vi "Temperature Controller Main.vi"() -> ()   [LabVIEW 2016, in "Desktop Application.lvlib"]
uses:
  Desktop Application.lvlib
  <vilib>/Skyline/Message/HTTP Wrapper/NI Skyline Message HTTP.lvclass
  <vilib>/Skyline/Configuration/Configuration HTTP_class/NI Skyline Configuration HTTP.lvclass
  <vilib>/Skyline/Configuration/Configuration HTTP_class/Open Configuration HTTP.vi
  <vilib>/Skyline/Message/HTTP Wrapper/Open (HTTP).vi
  <vilib>/Skyline/Message/NI Skyline Message.lvclass
  <vilib>/Skyline/Configuration/Configuration_class/NI Skyline Configuration.lvclass
panel:
  out "Heater State":bool
  in  "Low Limit":dbl
  in  "High Limit":dbl
  in  "Programatic Stop":bool
  out "CurrentTemperature":dbl(slide) scale=0.0..100.0
  out "Heater State Trend":i16(graph)
  out "Temperature Trend":T1(graph)
  # "Temperature Controller running on windows"
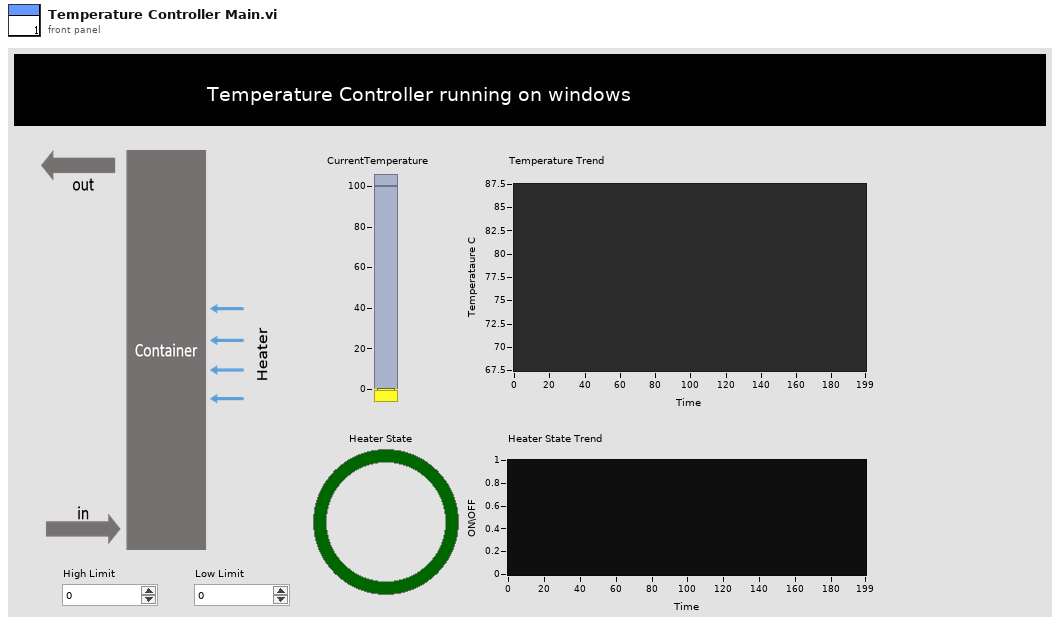
[diagram p1: front panel]
types:
  T1 = cluster{"Current Temp":dbl, "Low Set Point":dbl, "High Set Point":dbl}
  T2 = enum32{"invalid app kind", "Development System", "Run Time System", "Student Edition", "Embedded LabVIEW", "Evaluation", "Custom"}
  T3 = cluster{"Current Temp":dbl, "Low Set Point":dbl, "High Set Point":dbl}[]
  T4 = enum32{"Invalid", "Standard", "Closed", "Hidden", "Minimized", "Maximized"}
  T5 = cluster{"Core":cluster{"Current VI Reference":refnum<vi>, "Close Panel on Exit?":bool}, "High Set Point":dbl, "Low Set Point":dbl, "Current Temp":dbl, "Heater ON?":bool, "Skyline":refnum<class "NI Skyline Message HTTP.lvclass">, "SLconnected?":bool, "HTTP onfiguration":refnum<class "NI Skyline Configuration HTTP.lvclass">}
  T6 = cluster{"Current VI Reference":refnum<vi>, "Close Panel on Exit?":bool}
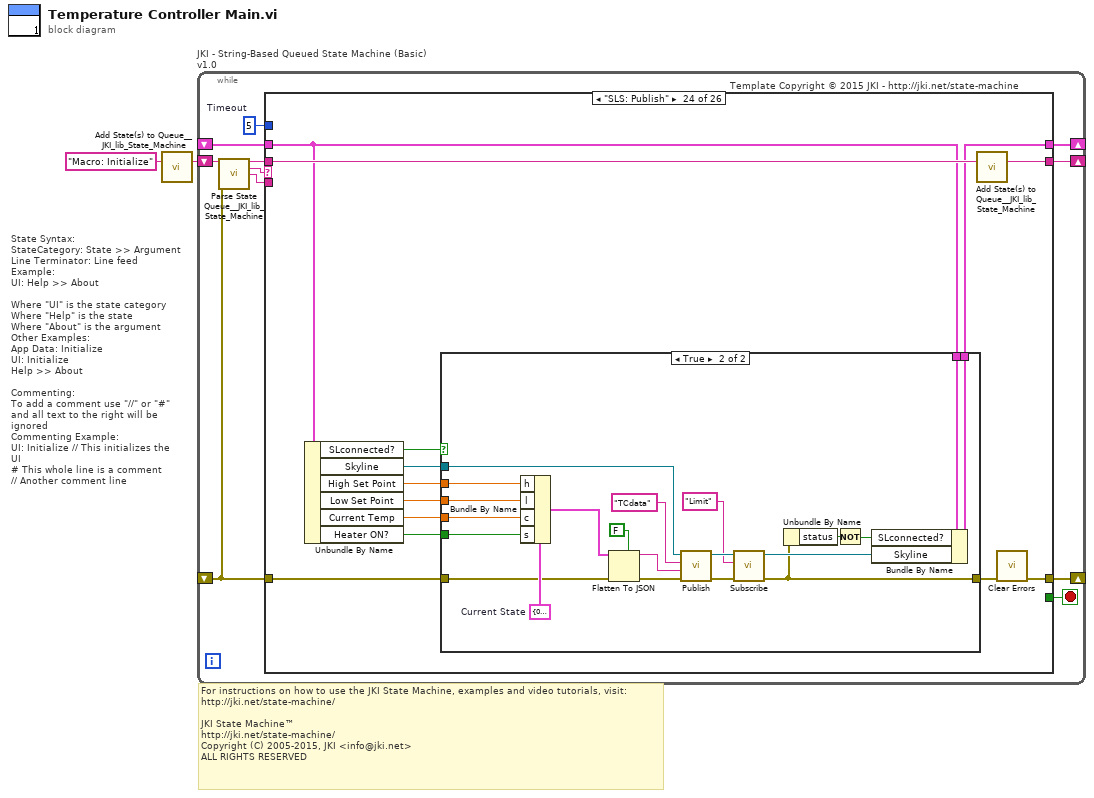
[diagram p0: block diagram]
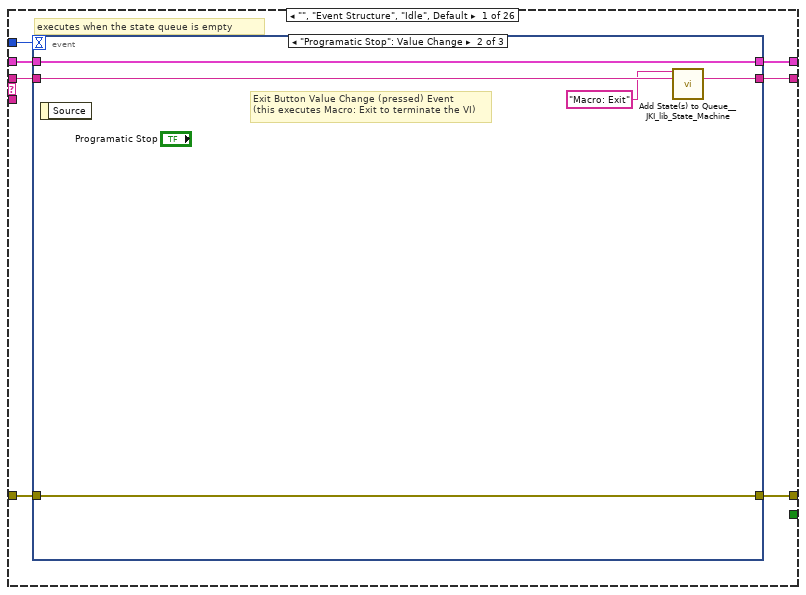
[diagram p2: hidden frame]
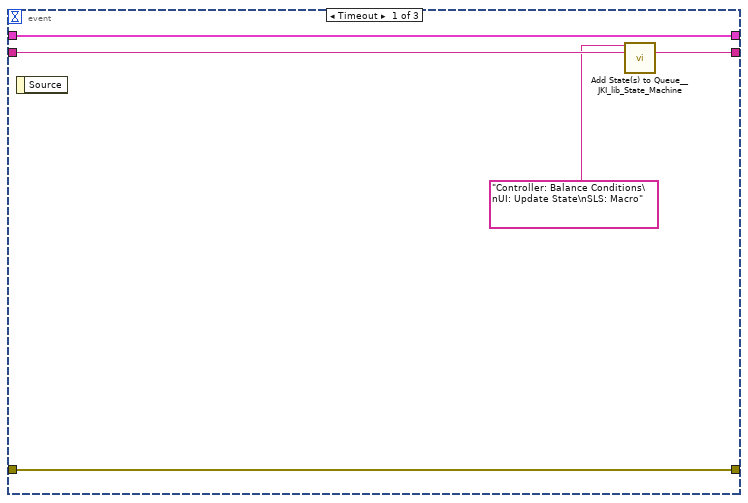
[diagram p3: hidden frame]
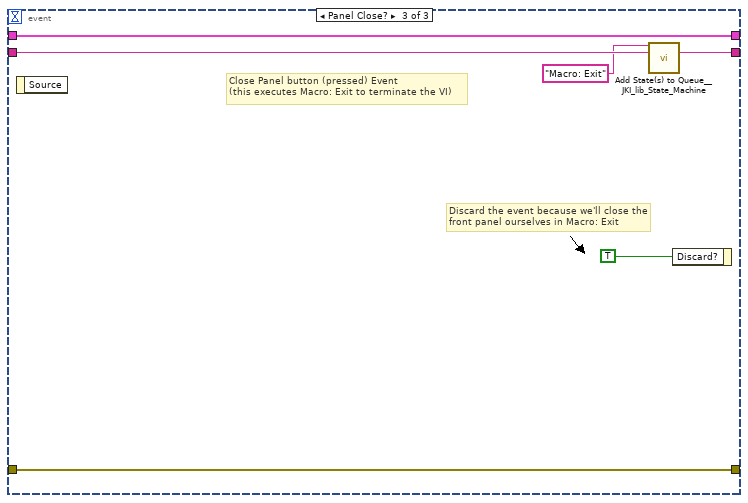
[diagram p4: hidden frame]
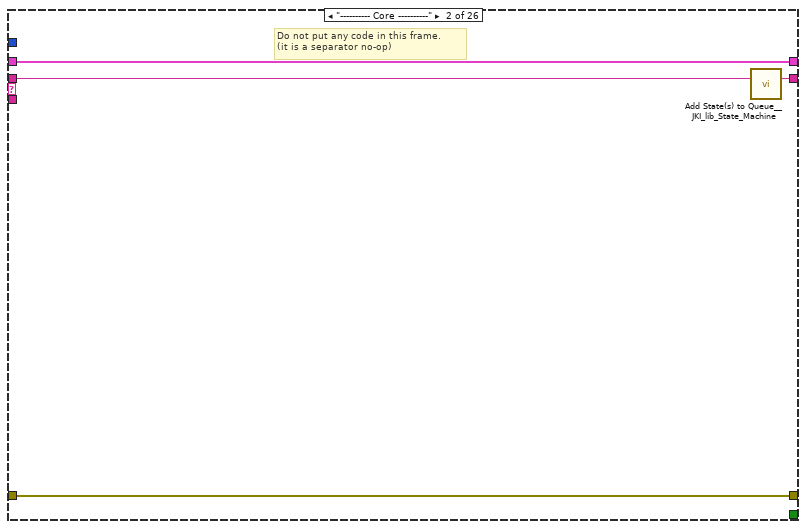
[diagram p5: hidden frame]
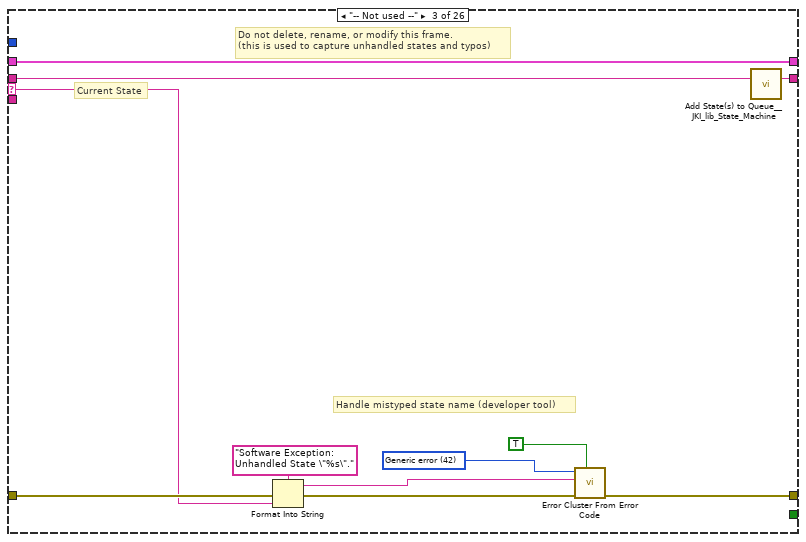
[diagram p6: hidden frame]
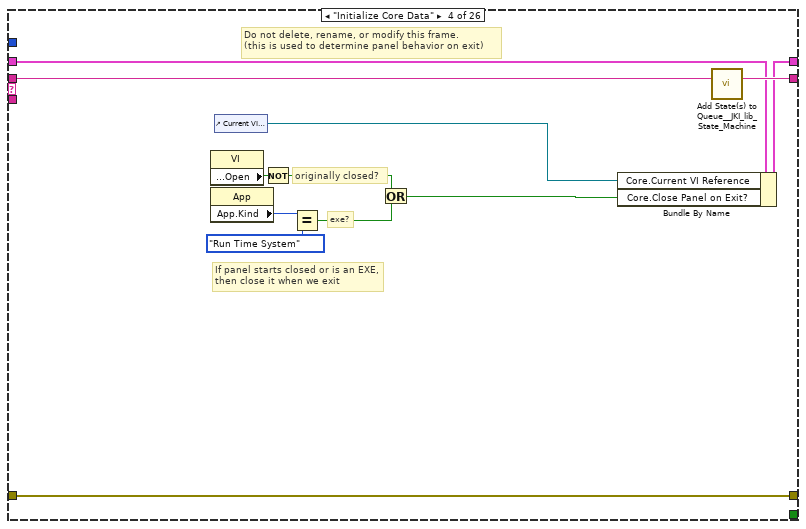
[diagram p7: hidden frame]
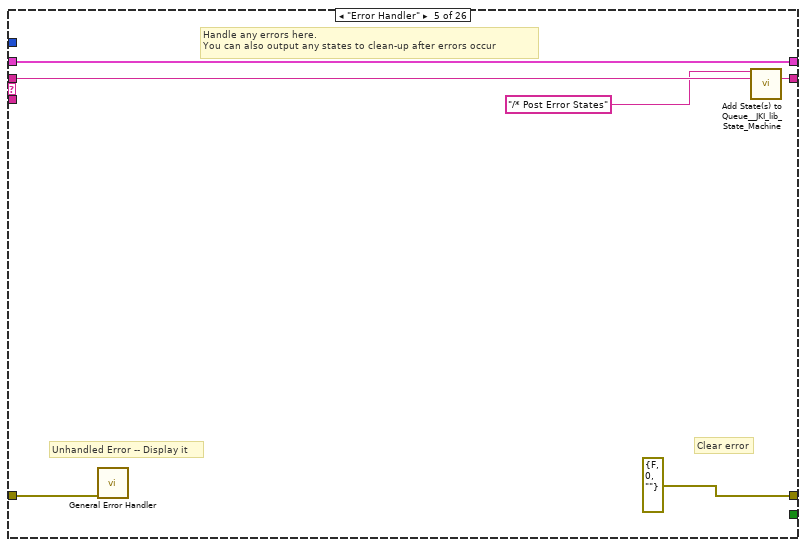
[diagram p8: hidden frame]
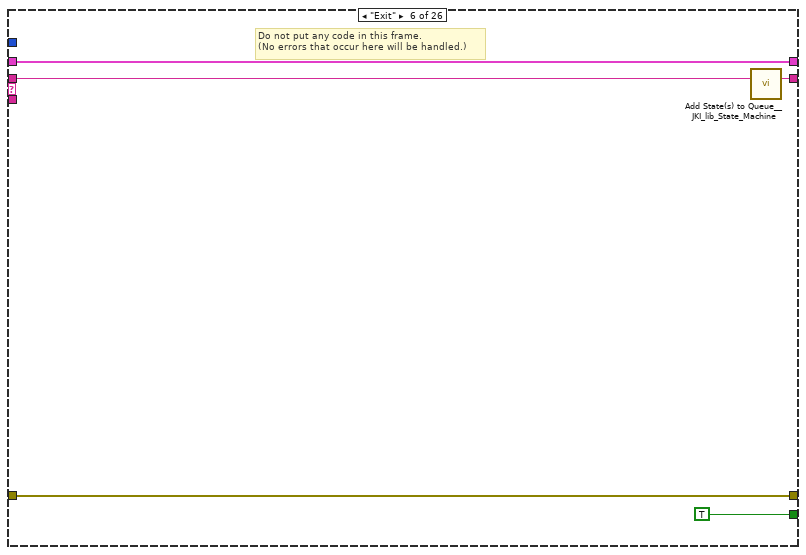
[diagram p9: hidden frame]
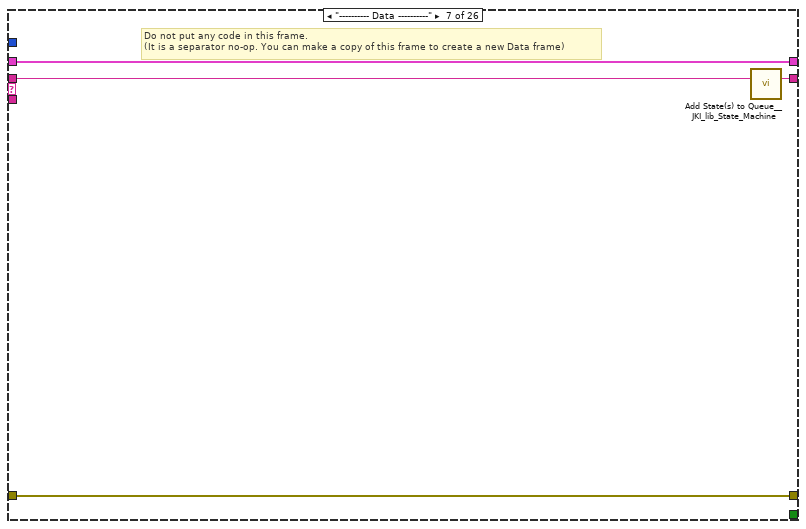
[diagram p10: hidden frame]
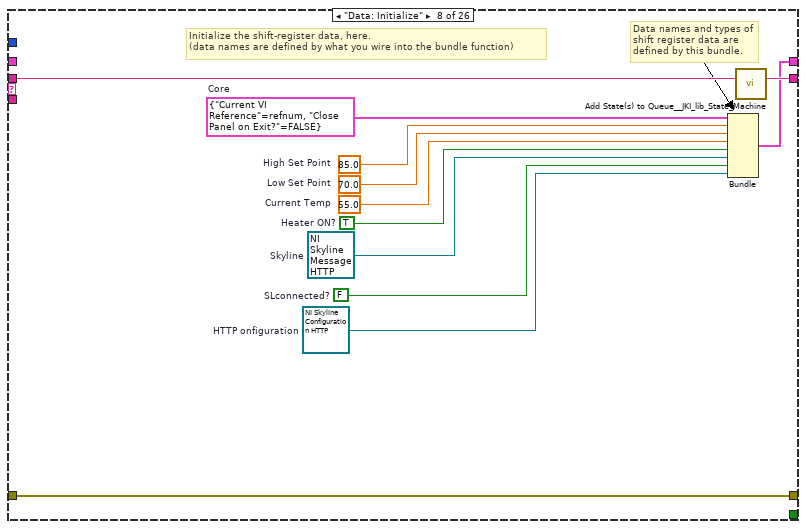
[diagram p11: hidden frame]
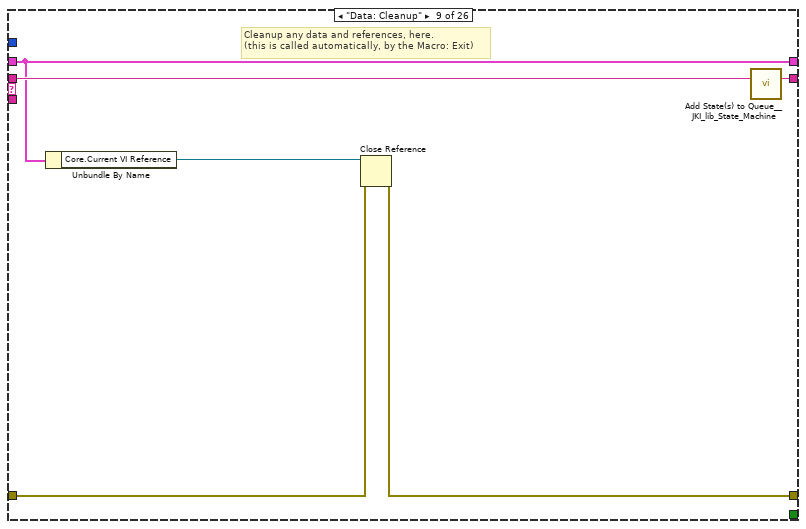
[diagram p12: hidden frame]
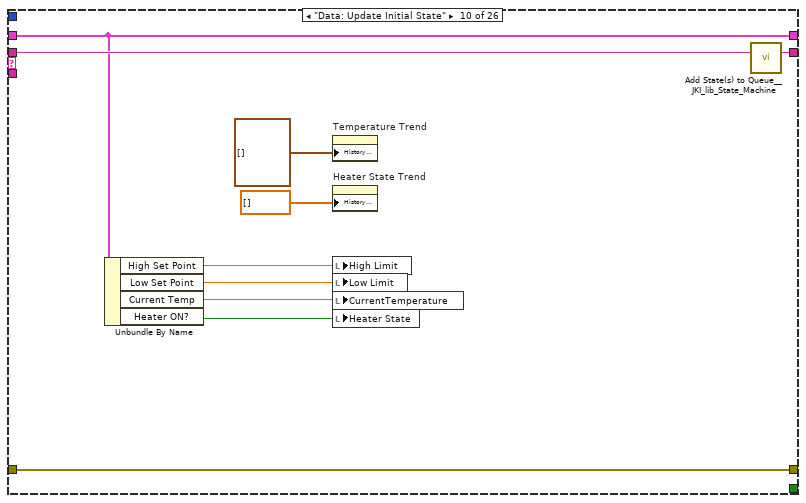
[diagram p13: hidden frame]
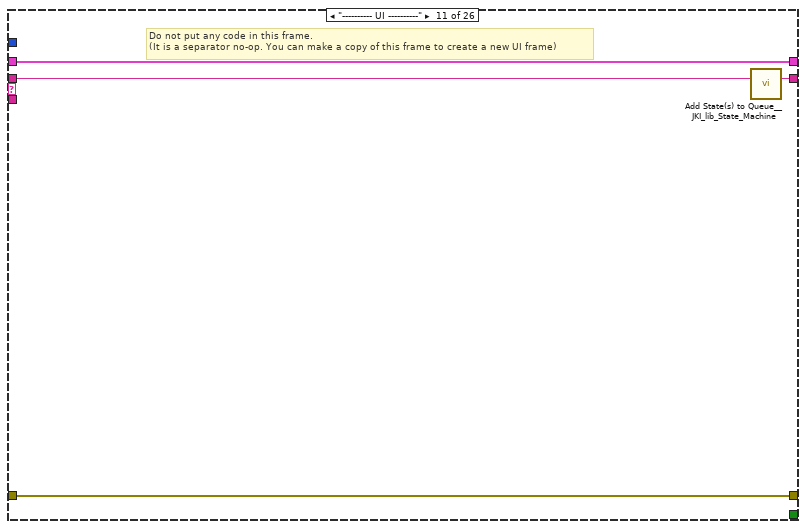
[diagram p14: hidden frame]
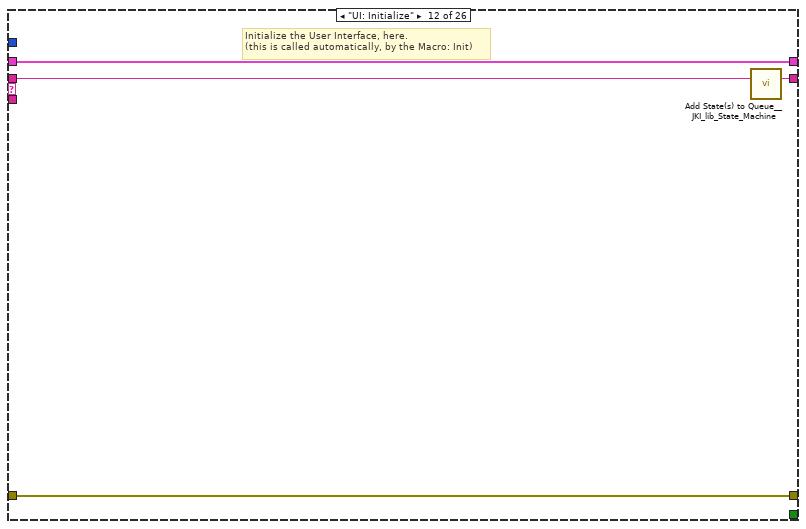
[diagram p15: hidden frame]
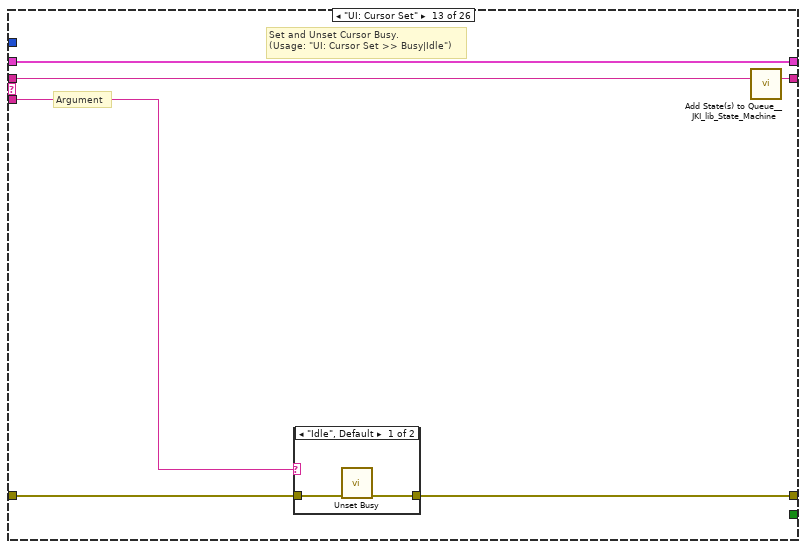
[diagram p16: hidden frame]
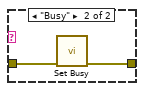
[diagram p17: hidden frame]
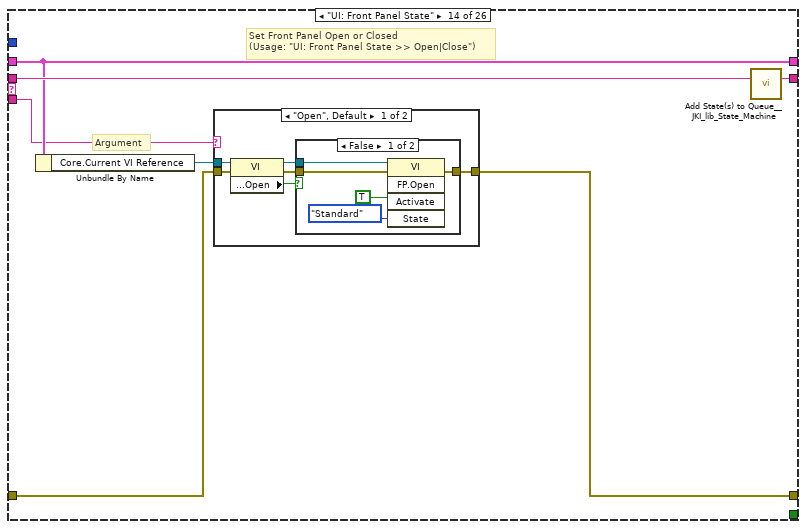
[diagram p18: hidden frame]
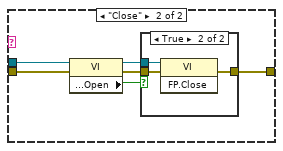
[diagram p20: hidden frame]
diagram:
  # "For instructions on how to use the JKI State Machine, examples and video tutorials, visit:\nhttp://jki.net/state-machine/\n\nJKI State Machine™\nhttp://jki.net/state-machine/\nCopyright (C) 2005-2015, JKI <info@jki.net>\nALL RIGHTS RESERVED"
  # "State Syntax:\nStateCategory: State >> Argument\nLine Terminator: Line feed\nExample:\nUI: Help >> About\n\nWhere \"UI\" is the state category\nWhere \"Help\" is the state\nWhere \"About\" is the argument\nOther Examples:\nApp Data: Initialize\nUI: Initialize\nHelp >> About\n\nCommenting:\nTo add a comment use \"//\" or \"#\" and all text to the right will be ignored\nCommenting Example:\nUI: Initialize // This initializes the UI\n# This whole line is a comment\n// Another comment line"
  n1 = call <vilib>:"Add State(s) to Queue__JKI_lib_State_Machine.vi"("State(s) in (\"\")"="Macro: Initialize") -> ("States Out"=w2:string)  [unwired: 14 in]
  n2 = while "JKI - String-Based Queued State Machine (Basic) v1.0" {
    shift-right: [w6] -> _
    shift-left: _ -> [w5]
    shift-right: [w9] -> _
    shift-left: _ -> [w3]
    shift-right: [w8] -> _
    shift-left: w2 -> [w10]
    stop <- w7 stop-if-true
    w4 = 5  # Timeout
    # "Template Copyright © 2015 JKI - http://jki.net/state-machine"
    n3 = call <vilib>:"Parse State Queue__JKI_lib_State_Machine.vi"("State Queue"=w10, "Error In (no error)"=w3) -> ("Remaining States"=w12:string, "Current State"=w13:string, "Arguments"=w11:string)  [unwired: 11 in]
    n4 = case shown="\"SLS: Publish\"" w13 {
      selector: w13 -> [_ _ w41 _ _ _ _ _ _ _ _ _ _ _ _ _ _ _ _ _ _ _ _ _ _ _]
      tunnel: w12 -> [w20 w40 w45 w63 w69 w74 w78 w90 w96 w106 w110 w114 w120 w131 w162 w167 w172 w177 w187 w191 w209 w211 w219 w246 w273 w299]
      tunnel: w11 -> [_ _ _ _ _ _ _ _ _ _ _ _ w115 w125 _ _ _ _ _ _ _ _ _ _ _ _]
      tunnel: w5 -> [w18 w37 w43 w54 w66 w72 w75 _ w91 w101 w107 w112 w118 w127 w160 w164 w169 w174 w184 w188 w204 w212 w216 w236 w274 w298]
      tunnel: [w17 w38 w47 w60 errorcluster {"status"=FALSE, "code"=0, "source"=""} ("error out") w71 w76 w87 w92 w104 w108 w111 w116 w128 w163 w165 w170 w175 w185 w189 w207 w210 w214 w239 w270 w295] -> w9
      tunnel: w3 -> [w16 w38 w46 w60 w65 w71 w76 w87 w93 w104 w108 w111 w117 w129 w163 w165 w170 w175 w185 w189 w207 w210 w218 w240 w275 w296]
      tunnel: [w19 w39 w44 w62 w68 w73 w77 w89 w95 w105 w109 w113 w119 w130 w161 w166 w171 w176 w186 w190 w208 w211 w219 w245 w273 w299] -> w8
      tunnel: [_ _ _ _ _ TRUE _ _ _ _ _ _ _ _ _ _ _ _ _ _ _ _ _ _ _ _] -> w7
      tunnel: [w15 w37 w43 w61 w66 w72 w75 w88 w91 w101 w107 w112 w118 w127 w160 w164 w169 w174 w184 w188 w203 w212 w217 w235 w274 w298] -> w6
      tunnel: w4 -> [w14 _ _ _ _ _ _ _ _ _ _ _ _ _ _ _ _ _ _ _ _ _ _ _ _ _]
      frame "", "Event Structure", "Idle", Default {
        # "executes when the state queue is empty"
        n5 = event shown="[1] \"Programatic Stop\": Value Change" {
          selector: _ -> [_ _ _]
          dyn-events: _ -> [_ _ _]
          timeout: w14 -> [_ _ _]
          tunnel: w20 -> [w25 w30 w36]
          tunnel: [w24 w29 w35] -> w19
          tunnel: w18 -> [w22 w27 w33]
          tunnel: [w23 w28 w34] -> w17
          tunnel: w16 -> [w23 w28 w34]
          tunnel: [w22 w27 w33] -> w15
          event Timeout {
            n6 = event-data() -> ()  [unwired: 1 in, 1 out]
            n7 = call <vilib>:"Add State(s) to Queue__JKI_lib_State_Machine.vi"("State(s) in Front (\"\")"="Controller: Balance Conditions\nUI: Update State\nSLS: Macro" ("State(s) in Front (\"\")"), "State(s) in (\"\")"=w25) -> ("States Out"=w24:string)  [unwired: 13 in]
          }
          event "Programatic Stop": Value Change {
            # "Exit Button Value Change (pressed) Event\n(this executes Macro: Exit to terminate the VI)"
            n8 = event-data() -> ()  [unwired: 1 in, 1 out]
            n9 = call <vilib>:"Add State(s) to Queue__JKI_lib_State_Machine.vi"("State(s) in Front (\"\")"="Macro: Exit", "State(s) in (\"\")"=w30) -> ("States Out"=w29:string)  [unwired: 13 in]
          }
          event Panel Close? {
            # "Discard the event because we'll close the front panel ourselves in Macro: Exit"
            # "Close Panel button (pressed) Event\n(this executes Macro: Exit to terminate the VI)"
            n10 = event-data() -> ()  [unwired: 1 in, 1 out]
            n11 = call <vilib>:"Add State(s) to Queue__JKI_lib_State_Machine.vi"("State(s) in Front (\"\")"="Macro: Exit", "State(s) in (\"\")"=w36) -> ("States Out"=w35:string)  [unwired: 13 in]
            n12 = event-data("Discard?"=TRUE) -> ()  [unwired: 1 in, 1 out]
          }
        }
      }
      frame "---------- Core ----------" {
        # "Do not put any code in this frame.\n(it is a separator no-op)"
        n13 = call <vilib>:"Add State(s) to Queue__JKI_lib_State_Machine.vi"("State(s) in (\"\")"=w40) -> ("States Out"=w39:string)  [unwired: 14 in]
      }
      frame "-- Not used --" {
        w50 = 42 items=["No error", "Argument error", "Memory is full", "Out of zone", "End of file", "File already open", "Generic file I/O error", "File not found", "File permission error", "Disk is full", "Duplicate path", "Too many files open", "System feature not enabled", "Resource file not found", "Cannot add resource", "Resource not found", "Image not found", "Image memory error", "Pen does not exist", "Config type invalid", "Config token not found", "Config parse error", "Config memory error", "Bad external code format", "Bad external code offset", "External code not present", "Null window", "Destroy window error", "Null menu", "Print aborted", "Bad print record", "Print driver error", "Windows error during printing", "Memory error during printing", "Print dialog error", "Generic print error", "Invalid device refnum", "Device not found", "Device parameter error", "Device unit error", "Cannot open device", "Device call aborted", "Generic error", "Cancelled by user", "Object ID too low", "Object ID too high", "Object not in heap", "Unknown heap", "Unknown object (invalid DefProc)", "Unknown object (DefProc not in table)", "Message out of range", "Invalid (null) method", "Unknown message", "Manager call not supported", "Bad address", "Network operation in progress", "Network operation timed out", "Connection is busy", "Network attribute not supported", "Network error", "Address in use", "System out of memory", "Connection aborted", "Connection refused", "Not connected", "Already connected", "Connection closed", "Initialization error (interapplication manager)", "Bad occurrence", "Wait on unbound occurrence handler", "Occurrence queue overflow", "Datalog type conflict", "Unused", "Unrecognized type (interapplication manager)", "Memory corrupt", "Failed to make temporary DLL", "Old CIN version", "Drag socket not found", "Failed to load drop-object", "Failed to register OLE object", "Failed to release OLE object", "Format specifier type mismatch", "Unknown format specifier", "Too few format specifiers", "Too many format specifiers", "Scan failed", "Newer CIN version", "Error converting to variant", "Runtime menu error", "Password tampered", "Variant attribute not found", "Incompatible variant data type", "Event data is not available", "Event Store is not present", "Occurrence is not found", "Event Queue is not created", "Event info is not available", "Refnum passed is NULL", "Error retrieving Class GUID", "Error retrieving CoClass GUID", "Error retrieving TypeLib GUID.", "Bad built application magic bytes.", "Specific driver is different from the specific driver associated with the Logical Name.", "There is no session opened to the class driver.", "Max Error", "MAX - Error with config objects", "MAX - Error loading configuration", "MAX - Group not supported"]
        # "Current State"
        # "Do not delete, rename, or modify this frame.\n(this is used to capture unhandled states and typos)"
        # "Handle mistyped state name (developer tool)"
        n14 = Format Into String(format string="Software Exception: Unhandled State \"%s\"." ("message"), error in=w46, w41) -> (resulting string=w49:string, error out=w48:errorcluster)  [unwired: 1 in]
        n15 = call <vilib>:"Error Cluster From Error Code.vi"("show call chain? (False)"=TRUE, "error in (no error)"=w48, "error message (\"\")"=w49, "error code (0)"=w50) -> ("error out"=w47:errorcluster)  [unwired: 5 in]
        n16 = call <vilib>:"Add State(s) to Queue__JKI_lib_State_Machine.vi"("State(s) in (\"\")"=w45) -> ("States Out"=w44:string)  [unwired: 14 in]
      }
      frame "Initialize Core Data" {
        # "Do not delete, rename, or modify this frame.\n(this is used to determine panel behavior on exit)"
        # "originally closed?"
        # "exe?"
        # "If panel starts closed or is an EXE, then close it when we exit"
        n17 = property class="VI"() -> ("Front Panel.Open"=w59:bool)  [unwired: 2 in, 2 out]
        n18 = property class="App"() -> ("App.Kind"=w58:T2)  [unwired: 2 in, 2 out]
        n19 = control-ref of="Current VI Reference"() -> (w52:refnum<vi>)
        n20 = Not(x=w59) -> (.not. x?=w56:bool)
        n21 = Equal?(x=w58, y=T2."Run Time System" ("Application:Kind")) -> (x = y?=w55:bool)
        n22 = Or(x=w56, y=w55) -> (x .or. y?=w53:bool)
        n23 = Bundle By Name(cluster=w54, "Core.Current VI Reference"=w52, "Core.Close Panel on Exit?"=w53) -> (w61:T5)
        n24 = call <vilib>:"Add State(s) to Queue__JKI_lib_State_Machine.vi"("State(s) in (\"\")"=w63) -> ("States Out"=w62:string)  [unwired: 14 in]
      }
      frame "Error Handler" {
        # "Unhandled Error -- Display it"
        # "Handle any errors here.\nYou can also output any states to clean-up after errors occur"
        # "Clear error"
        n25 = call <vilib>:"General Error Handler.vi"("error in (no error)"=w65) -> ()  [unwired: 10 in, 5 out]
        n26 = call <vilib>:"Add State(s) to Queue__JKI_lib_State_Machine.vi"("State(s) in Front (\"\")"="/* Post Error States", "State(s) in (\"\")"=w69) -> ("States Out"=w68:string)  [unwired: 13 in]
      }
      frame "Exit" {
        # "Do not put any code in this frame.\n(No errors that occur here will be handled.)"
        n27 = call <vilib>:"Add State(s) to Queue__JKI_lib_State_Machine.vi"("State(s) in (\"\")"=w74) -> ("States Out"=w73:string)  [unwired: 14 in]
      }
      frame "---------- Data ----------" {
        # "Do not put any code in this frame.\n(It is a separator no-op. You can make a copy of this frame to create a new Data frame)"
        n28 = call <vilib>:"Add State(s) to Queue__JKI_lib_State_Machine.vi"("State(s) in (\"\")"=w78) -> ("States Out"=w77:string)  [unwired: 14 in]
      }
      frame "Data: Initialize" {
        w79 = refnum<class "NI Skyline Configuration HTTP.lvclass"> refnum  # HTTP onfiguration
        w80 = FALSE  # SLconnected?
        w81 = refnum<class "NI Skyline Message HTTP.lvclass"> refnum  # Skyline
        w82 = TRUE  # Heater ON?
        w83 = 55.0  # Current Temp
        w84 = 70.0  # Low Set Point
        w85 = 85.0  # High Set Point
        w86 = T6 {"Current VI Reference"=refnum, "Close Panel on Exit?"=FALSE}  # Core
        # "Data names and types of shift register data are defined by this bundle."
        # "Initialize the shift-register data, here.\n(data names are defined by what you wire into the bundle function)"
        n29 = Bundle("Core"=w86, "High Set Point"=w85, "Low Set Point"=w84, "Current Temp"=w83, "Heater ON?"=w82, "Skyline"=w81, "SLconnected?"=w80, "HTTP onfiguration"=w79) -> (w88:T5)  [unwired: 1 in]
        n30 = call <vilib>:"Add State(s) to Queue__JKI_lib_State_Machine.vi"("State(s) in (\"\")"=w90) -> ("States Out"=w89:string)  [unwired: 14 in]
      }
      frame "Data: Cleanup" {
        # "Cleanup any data and references, here.\n(this is called automatically, by the Macro: Exit)"
        n31 = Unbundle By Name(w91) -> ("Core.Current VI Reference"=w94:refnum<vi>)
        n32 = Close Reference(reference=w94, error in (no error)=w93) -> (error out=w92:errorcluster)
        n33 = call <vilib>:"Add State(s) to Queue__JKI_lib_State_Machine.vi"("State(s) in (\"\")"=w96) -> ("States Out"=w95:string)  [unwired: 14 in]
      }
      frame "Data: Update Initial State" {
        n34 = Unbundle By Name(w101) -> ("High Set Point"=w100:dbl, "Low Set Point"=w99:dbl, "Current Temp"=w97:dbl, "Heater ON?"=w98:bool)
        n35 = property on="Temperature Trend" class="WFChart (strict)"("History Data"=T3 []) -> ()  [unwired: 2 in, 2 out]
        n36 = property on="Heater State Trend" class="WFChart (strict)"("History Data"=dbl[] []) -> ()  [unwired: 2 in, 2 out]
        n37 = local write "High Limit"(w100) -> ()
        n38 = local write "Low Limit"(w99) -> ()
        n39 = local write "CurrentTemperature"(w97) -> ()
        n40 = local write "Heater State"(w98) -> ()
        n41 = call <vilib>:"Add State(s) to Queue__JKI_lib_State_Machine.vi"("State(s) in (\"\")"=w106) -> ("States Out"=w105:string)  [unwired: 14 in]
      }
      frame "---------- UI ----------" {
        # "Do not put any code in this frame.\n(It is a separator no-op. You can make a copy of this frame to create a new UI frame)"
        n42 = call <vilib>:"Add State(s) to Queue__JKI_lib_State_Machine.vi"("State(s) in (\"\")"=w110) -> ("States Out"=w109:string)  [unwired: 14 in]
      }
      frame "UI: Initialize" {
        # "Initialize the User Interface, here.\n(this is called automatically, by the Macro: Init)"
        n43 = call <vilib>:"Add State(s) to Queue__JKI_lib_State_Machine.vi"("State(s) in (\"\")"=w114) -> ("States Out"=w113:string)  [unwired: 14 in]
      }
      frame "UI: Cursor Set" {
        # "Argument"
        # "Set and Unset Cursor Busy.\n(Usage: \"UI: Cursor Set >> Busy|Idle\")"
        n44 = case shown="\"Idle\", Default" w115 {
          tunnel: w117 -> [w122 w124]
          tunnel: [w121 w123] -> w116
          frame "Idle", Default {
            n45 = call <vilib>:"Unset Busy.vi"("error in (no error)"=w122) -> ("error out"=w121:errorcluster)  [unwired: 10 in]
          }
          frame "Busy" {
            n46 = call <vilib>:"Set Busy.vi"("error in (no error)"=w124) -> ("error out"=w123:errorcluster)  [unwired: 9 in, 1 out]
          }
        }
        n47 = call <vilib>:"Add State(s) to Queue__JKI_lib_State_Machine.vi"("State(s) in (\"\")"=w120) -> ("States Out"=w119:string)  [unwired: 14 in]
      }
      frame "UI: Front Panel State" {
        # "Argument"
        # "Set Front Panel Open or Closed\n(Usage: \"UI: Front Panel State >> Open|Close\")"
        n48 = Unbundle By Name(w127) -> ("Core.Current VI Reference"=w126:refnum<vi>)
        n49 = case shown="\"Open\", Default" w125 {
          tunnel: w129 -> [w135 w148]
          tunnel: [w137 w149] -> w128
          tunnel: w126 -> [w136 w146]
          frame "Open", Default {
            n50 = property class="VI"(reference=w136, error in=w135) -> (reference out=w133:refnum<vi>, error out=w134:errorcluster, "Front Panel.Open"=w132:bool)
            n51 = case shown="False" w132 {
              tunnel: [w140 w143] -> w137
              tunnel: w134 -> [w139 w143]
              tunnel: w133 -> [w138 _]
              frame False {
                n52 = invoke class="VI" method="FP.Open"(reference=w138, error in=w139, "Activate"=TRUE, "State"=T4."Standard") -> (error out=w140:errorcluster)  [unwired: 1 in, 4 out]
              }
              frame True {
              }
            }
          }
          frame "Close" {
            n53 = property class="VI"(reference=w146, error in=w148) -> (reference out=w145:refnum<vi>, error out=w147:errorcluster, "Front Panel.Open"=w144:bool)
            n54 = case shown="True" w144 {
              tunnel: [w150 w153] -> w149
              tunnel: w147 -> [w150 w152]
              tunnel: w145 -> [_ w151]
              frame False {
              }
              frame True {
                n55 = invoke class="VI" method="FP.Close"(reference=w151, error in=w152) -> (error out=w153:errorcluster)  [unwired: 1 in, 2 out]
              }
            }
          }
        }
        n56 = call <vilib>:"Add State(s) to Queue__JKI_lib_State_Machine.vi"("State(s) in (\"\")"=w131) -> ("States Out"=w130:string)  [unwired: 14 in]
      }
      frame "UI: Update State" {
        n57 = Unbundle By Name(w160) -> ("High Set Point"=w155:dbl, "Low Set Point"=w156:dbl, "Current Temp"=w157:dbl, "Heater ON?"=w158:bool)
        "CurrentTemperature" <- w157
        "Heater State" <- w158
        n58 = Boolean To (0,1)(Boolean=w158) -> (0, 1=→"Heater State Trend":i16)
        n59 = Bundle("Current Temp"=w157, "Low Set Point"=w156, "High Set Point"=w155) -> (→"Temperature Trend":T1)  [unwired: 1 in]
        n60 = call <vilib>:"Add State(s) to Queue__JKI_lib_State_Machine.vi"("State(s) in (\"\")"=w162) -> ("States Out"=w161:string)  [unwired: 14 in]
      }
      frame "---------- Macro ----------" {
        # "Do not put any code in this frame.\n(It is a separator no-op. You can make a copy of this frame to create a new Macro frame)"
        n61 = call <vilib>:"Add State(s) to Queue__JKI_lib_State_Machine.vi"("State(s) in (\"\")"=w167) -> ("States Out"=w166:string)  [unwired: 14 in]
      }
      frame "Macro: Initialize" {
        w168 = "Data: Initialize\nInitialize Core Data\nUI: Initialize\nUI: Front Panel State >> Open\nData: Update Initial State\nUI: Update State\nSLS: Open"  # Data: Initialize Initialize Core Data UI: Initialize UI: Front Panel State >> Open Data: Update Initial State UI: Update State SLS: Open
        # "Initialization Macro\n(This is called once, when the VI starts)"
        n62 = call <vilib>:"Add State(s) to Queue__JKI_lib_State_Machine.vi"("State(s) in Front (\"\")"=w168, "State(s) in (\"\")"=w172) -> ("States Out"=w171:string)  [unwired: 13 in]
      }
      frame "SLS: Macro" {
        # "Initialization Macro\n(This is called once, when the VI starts)"
        n63 = call <vilib>:"Add State(s) to Queue__JKI_lib_State_Machine.vi"("State(s) in Front (\"\")"="SLS: Open\nSLS: Publish\nSLS: Read", "State(s) in (\"\")"=w177) -> ("States Out"=w176:string)  [unwired: 13 in]
      }
      frame "Macro: Exit" {
        # "Exit Macro\n(This is called once, when the VI exits)"
        n64 = Unbundle By Name(w184) -> ("Core.Close Panel on Exit?"=w183:bool)
        n65 = Select(t="UI: Front Panel State >> Close", s=w183, f="") -> (s? t:f=w180:string)
        n66 = call <vilib>:"Add State(s) to Queue__JKI_lib_State_Machine.vi"("State(s) in (\"\")"=w180, "State(s) at Back (\"\")"="Data: Cleanup\nSLS: Close\nExit") -> ("States Out"=w178:string)  [unwired: 13 in]
        n67 = call <vilib>:"Add State(s) to Queue__JKI_lib_State_Machine.vi"("State(s) in Front (\"\")"=w178, "State(s) in (\"\")"=w187) -> ("States Out"=w186:string)  [unwired: 13 in]
      }
      frame "---------- Functions ----------" {
        # "Template Separator\n(You can make a copy of, or modify, this frame)"
        n68 = call <vilib>:"Add State(s) to Queue__JKI_lib_State_Machine.vi"("State(s) in (\"\")"=w191) -> ("States Out"=w190:string)  [unwired: 14 in]
      }
      frame "Controller: Balance Conditions" {
        n69 = Unbundle By Name(w204) -> ("Heater ON?"=w196:bool, "Current Temp"=w194:dbl)
        n70 = Max & Min(x="High Limit", y="Low Limit") -> (max(x,y)=w202:dbl, min(x,y)=w193:dbl)
        n71 = Less?(x=w194, y=w193) -> (x < y?=w192:bool)
        n72 = In Range and Coerce(upper limit=w202, x=w194, lower limit=w193) -> (In Range?=w197:bool)  [unwired: 1 out]
        n73 = Increment(x=w194) -> (x+1=w200:dbl)
        n74 = Decrement(x=w194) -> (x-1=w201:dbl)
        n75 = Select(t=w196, s=w197, f=w192) -> (s? t:f=w195:bool)
        n76 = Select(t=w200, s=w195, f=w201) -> (s? t:f=w199:dbl)
        n77 = Bundle By Name(cluster=w204, "High Set Point"=w202, "Low Set Point"=w193, "Heater ON?"=w195, "Current Temp"=w199) -> (w203:T5)
        n78 = Wait (ms)(milliseconds to wait=u32 300) -> ()  [unwired: 1 out]
        n79 = call <vilib>:"Add State(s) to Queue__JKI_lib_State_Machine.vi"("State(s) in (\"\")"=w209) -> ("States Out"=w208:string)  [unwired: 14 in]
      }
      frame "----------System Link Service----------" {
      }
      frame "SLS: Open" {
        n80 = Unbundle By Name(w216) -> ("SLconnected?"=w213:bool)
        n81 = case shown="True" w213 {
          tunnel: w218 -> [w231 w232]
          tunnel: [w229 w233] -> w217
          tunnel: w216 -> [w228 w233]
          tunnel: [w227 w232] -> w215
          frame False {
            n82 = call-poly <vilib>:"Open Configuration.vi"("error in (no error)"=w231, "password"="q", "username"="admin", "server url"="http://localhost:80") -> ("error out"=w223:errorcluster, "HTTP configuration out"=w224:refnum<class "NI Skyline Configuration HTTP.lvclass">)  [unwired: 6 in]
            n83 = call-poly <vilib>:"Open.vi"("configuration"=w224, "error in (no error)"=w223) -> ("error out"=w227:errorcluster, "message http out"=w230:refnum<class "NI Skyline Message HTTP.lvclass">)  [unwired: 8 in]
            n84 = Unbundle By Name(w227) -> ("status"=w226:bool)
            n85 = Not(x=w226) -> (.not. x?=w225:bool)
            n86 = Bundle By Name(cluster=w228, "HTTP onfiguration"=w224, "SLconnected?"=w225, "Skyline"=w230) -> (w229:T5)
          }
          frame True {
          }
        }
        n87 = call <vilib>:"Clear Errors.vi"("error in (no error)"=w215) -> ("error out"=w214:errorcluster)  [unwired: 5 in, 1 out]
      }
      frame "SLS: Publish" {
        n88 = Unbundle By Name(w236) -> ("SLconnected?"=w234:bool, "Skyline"=w237:refnum<class "NI Skyline Message HTTP.lvclass">, "High Set Point"=w244:dbl, "Low Set Point"=w243:dbl, "Current Temp"=w242:dbl, "Heater ON?"=w241:bool)
        n89 = case shown="True" w234 {
          tunnel: w244 -> [_ w268]
          tunnel: w243 -> [_ w267]
          tunnel: w242 -> [_ w266]
          tunnel: w241 -> [_ w265]
          tunnel: w240 -> [w248 w263]
          tunnel: [w248 w250] -> w238
          tunnel: w237 -> [_ w260]
          tunnel: w236 -> [w247 w259]
          tunnel: [w247 w258] -> w235
          frame False {
          }
          frame True {
            w269 = cluster{"h":dbl, "l":dbl, "c":dbl, "s":bool} {"h"=0.0, "l"=0.0, "c"=0.0, "s"=FALSE}  # Current State
            n90 = Bundle By Name(cluster=w269, "h"=w268, "l"=w267, "c"=w266, "s"=w265) -> (w264:cluster{"h":dbl, "l":dbl, "c":dbl, "s":bool})
            n91 = Flatten To JSON(enable LabVIEW extensions? (T)=FALSE, anything=w264, error in (no error)=w263) -> (JSON string=w257:string, 11:w261:errorcluster)
            n92 = call-dynamic "Publish.vi"("error in (no error)"=w261, "message"=w257, "topic"="TCdata", "message http"=w260) -> ("error out"=w251:errorcluster, "message http out"=w253:refnum<class "NI Skyline Message HTTP.lvclass">)  [unwired: 6 in]
            n93 = call-dynamic "Subscribe.vi"("error in (no error)"=w251, "topic"="Limit", "message http"=w253) -> ("error out"=w250:errorcluster, "message http out"=w252:refnum<class "NI Skyline Message HTTP.lvclass">)  [unwired: 7 in]
            n94 = Unbundle By Name(w250) -> ("status"=w255:bool)
            n95 = Not(x=w255) -> (.not. x?=w254:bool)
            n96 = Bundle By Name(cluster=w259, "SLconnected?"=w254, "Skyline"=w252) -> (w258:T5)
          }
        }
        n97 = call <vilib>:"Add State(s) to Queue__JKI_lib_State_Machine.vi"("State(s) in (\"\")"=w246) -> ("States Out"=w245:string)  [unwired: 14 in]
        n98 = call <vilib>:"Clear Errors.vi"("error in (no error)"=w238) -> ("error out"=w239:errorcluster)  [unwired: 5 in, 1 out]
      }
      frame "SLS: Read" {
        n99 = Unbundle By Name(w274) -> ("SLconnected?"=w271:bool, "Skyline"=w272:refnum<class "NI Skyline Message HTTP.lvclass">)
        n100 = case shown="True" w271 {
          tunnel: w275 -> [w276 w284]
          tunnel: w272 -> [_ w283]
          tunnel: [w276 w277] -> w270
          frame False {
          }
          frame True {
            n101 = call-dynamic "Read.vi"("error in (no error)"=w284, "timeout milliseconds (100)"=100, "message http"=w283) -> ("error out"=w278:errorcluster, "message"=w279:string, "topic"=w280:string, "dequeue status"=w281:bool)  [unwired: 4 in, 1 out]
            n102 = case shown="True" w281 {
              tunnel: w280 -> [_ _]
              tunnel: w279 -> [_ w290]
              tunnel: w278 -> [w285 w292]
              tunnel: [w285 w291] -> w277
              frame False {
              }
              frame True {
                w289 = cluster{"high":dbl, "low":dbl} {"high"=0.0, "low"=0.0}  # limit
                n103 = Unflatten From JSON(JSON string=w290, type and defaults=w289, error in (no error)=w292) -> (value=w288:cluster{"high":dbl, "low":dbl}, error out=w291:errorcluster)  [unwired: 4 in]
                n104 = Unbundle(w288) -> ("high"=w287:dbl, "low"=w286:dbl)
                n105 = local write "High Limit"(w287) -> ()
                n106 = local write "Low Limit"(w286) -> ()
              }
            }
          }
        }
      }
      frame "SLS: Close" {
        n107 = Unbundle By Name(w298) -> ("HTTP onfiguration"=w293:refnum<class "NI Skyline Configuration HTTP.lvclass">, "SLconnected?"=w294:bool, "Skyline"=w297:refnum<class "NI Skyline Message HTTP.lvclass">)
        n108 = case shown="True" w294 {
          tunnel: w297 -> [_ w303]
          tunnel: w296 -> [w300 w304]
          tunnel: [w300 w306] -> w295
          tunnel: w293 -> [_ w308]
          frame False {
          }
          frame True {
            n109 = call-dynamic "Unsubscribe.vi"("error in (no error)"=w304, "topic"="Limit", "message http"=w303) -> ("error out"=w301:errorcluster, "message http out"=w302:refnum<class "NI Skyline Message HTTP.lvclass">)  [unwired: 7 in]
            n110 = call-dynamic "Close.vi"("error in (no error)"=w301, "message http"=w302) -> ("error out"=w307:errorcluster)  [unwired: 9 in]
            n111 = call-dynamic "Close Configuration.vi"("error in (no error)"=w307, "HTTP configuration in"=w308) -> ("error out"=w306:errorcluster)  [unwired: 9 in]
          }
        }
      }
    }
  }
